vi "Generate Packet Identifier.vi"() -> (2 "Packet Identifier":u16 format="%04x")   [LabVIEW 2013, in "MQTT_Control_Packets.lvlib" / "ControlPacket.lvclass"]
uses:
  ControlPacket.lvclass
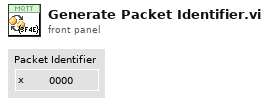
[diagram p1: front panel]
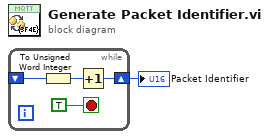
[diagram p0: block diagram]
diagram:
  n1 = while {
    shift-right: [w4] -> w1
    shift-left: _ -> [w3]
    stop <- TRUE stop-if-true
    n2 = To Unsigned Word Integer(number=w3) -> (unsigned 16bit integer=w2:u16)
    n3 = Increment(x=w2) -> (x+1=w4:u16)
  }
  "Packet Identifier" <- w1
